vi "Player Info.vi"(11 "64 in":refnum<class "Border.lvclass">) -> (0 "Defeat Speech":string, 1 "Victory Speech":string, 2 "Name":string, 3 "64 out":refnum<class "Border.lvclass">)   [LabVIEW 2015, in "Border.lvclass"]
uses:
  Border.lvclass
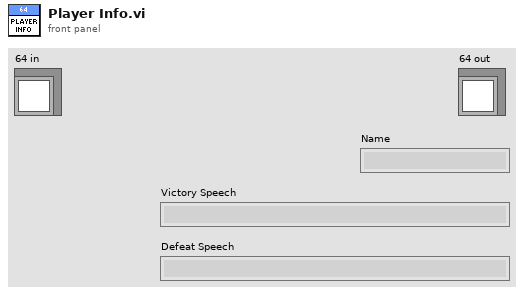
[diagram p1: front panel]
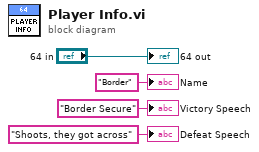
[diagram p0: block diagram]
diagram:
  "64 out" <- "64 in"
  "Name" <- "Border" ("Name")
  "Victory Speech" <- "Border Secure" ("Victory Speech")
  "Defeat Speech" <- "Shoots, they got across" ("Defeat Speech")
